vi "Temp Array Gen BAP3B.vi"(8 "error in (no error)":errorcluster, 11 "Temperature Control Parameters":T1={"Start Temp"=0.0, "Temp Step"=5.0, "End Temp"=0.0} {"End Temp" format="%.2f"; "Temp Step" format="%.2f"; "Start Temp" format="%.2f"}) -> (0 "error out":errorcluster, 1 "Temperature Control Parameters Out":T1={"Start Temp"=0.0, "Temp Step"=5.0, "End Temp"=0.0} {"End Temp" format="%.2f"; "Temp Step" format="%.2f"; "Start Temp" format="%.2f"}, 2 "N Temps":i32=6, 3 "Temp Array":dbl[](array[numeric]), 4 "Warning":bool=TRUE)   [LabVIEW 2014]
doc: "Temp Array Gen\n\nCreates an array of temperature given the starting, step, end temperature. This should return an array and the number of temperatures. Takes in consideration inverted limits and steps of zero.\n\nBeverly Abadines\nPHY 350 \nBAP3B"
uses:
  typedefs/temp control params.ctl
panel:
  # "Temp Array Gen"
  # "Beverly Abadines\nPhys 350\nBAP3B"
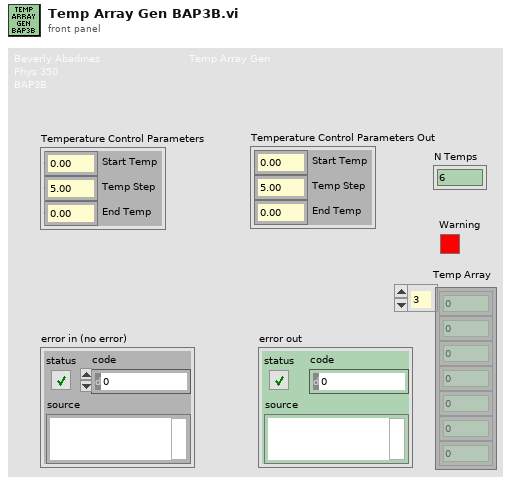
[diagram p1: front panel]
types:
  T1 = typedef "temp control params.ctl" = cluster{"Start Temp":dbl, "Temp Step":dbl, "End Temp":dbl}
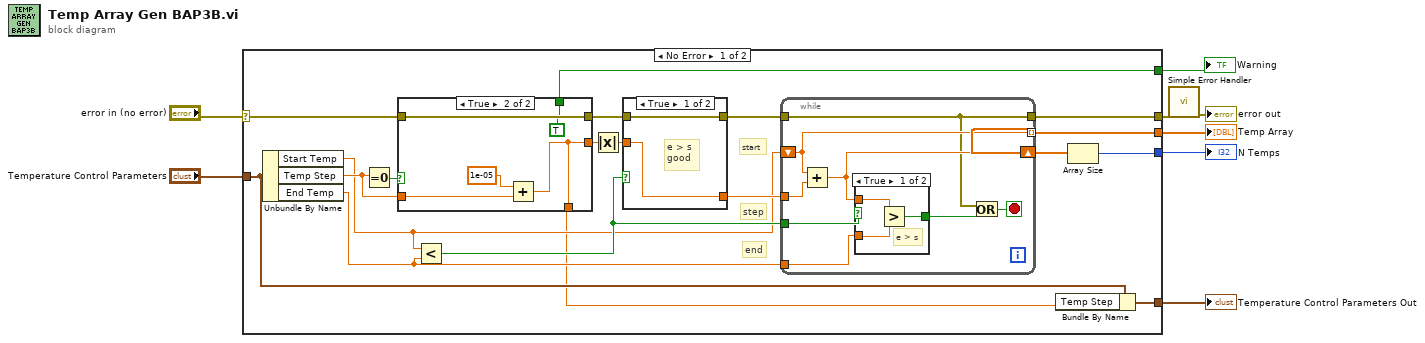
[diagram p0: block diagram]
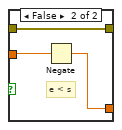
[diagram p2: hidden frame]
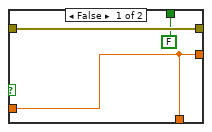
[diagram p3: hidden frame]
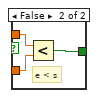
[diagram p4: hidden frame]
diagram:
  n1 = case shown="No Error" "error in (no error)" {
    selector: "error in (no error)" -> [w19 w54]
    tunnel: [w16 w54] -> w5
    tunnel: "Temperature Control Parameters" -> [w11 _]
    tunnel: [w18 _] -> w7
    tunnel: [w17 _] -> w6
    tunnel: [w12 _] -> w2
    tunnel: [w9 _] -> w1
    frame No Error {
      # "end"
      # "step"
      # "start"
      n2 = Unbundle By Name(w11) -> ("Start Temp"=w13:dbl, "Temp Step"=w21:dbl, "End Temp"=w14:dbl)
      n3 = Equal To 0?(x=w21) -> (x = 0?=w20:bool)
      n4 = case shown="True" w20 {
        tunnel: w21 -> [w33 w39]
        tunnel: [w33 w36] -> w22
        tunnel: w19 -> [w34 w37]
        tunnel: [w34 w37] -> w25
        tunnel: [w33 w36] -> w10
        tunnel: [FALSE TRUE] -> w9
        frame False {
        }
        frame True {
          n5 = Add(x=1e-05, y=w39) -> (x+y=w36:dbl)
        }
      }
      n6 = Less?(x=w13, y=w14) -> (x < y?=w24:bool)
      n7 = Absolute Value(x=w22) -> (abs(x)=w23:dbl)
      n8 = case shown="True" w24 {
        tunnel: w23 -> [w28 w31]
        tunnel: [w28 w30] -> w15
        tunnel: w25 -> [w27 w29]
        tunnel: [w27 w29] -> w26
        frame True {
          # "e > s \ngood"
        }
        frame False {
          # "e < s"
          n9 = Negate(x=w31) -> (-x=w30:dbl)
        }
      }
      n10 = while {
        shift-right: [w45] -> _
        shift-left: w13 -> [w47]
        tunnel: [w47] -> w18 mode=indexing
        tunnel: w14 -> [w44]
        tunnel: w15 -> [w46]
        tunnel: w24 -> [w43]
        tunnel: w26 -> [w41]
        tunnel: [w41] -> w16
        stop <- w40 stop-if-true
        n11 = Add(x=w47, y=w46) -> (x+y=w45:dbl)
        n12 = case shown="True" w43 {
          tunnel: w45 -> [w50 w53]
          tunnel: w44 -> [w49 w52]
          tunnel: [w48 w51] -> w42
          frame True {
            # "e > s"
            n13 = Greater?(x=w50, y=w49) -> (0:w48:bool)
          }
          frame False {
            # "e < s"
            n14 = Less?(x=w53, y=w52) -> (x < y?=w51:bool)
          }
        }
        n15 = Or(x=w41, y=w42) -> (x .or. y?=w40:bool)
      }
      n16 = Bundle By Name(cluster=w11, "Temp Step"=w10) -> (w12:T1)
      n17 = Array Size(array=w18) -> (size(s)=w17:i32)
    }
    frame Error {
    }
  }
  "N Temps" <- w6
  "Temp Array" <- w7
  "Temperature Control Parameters Out" <- w2
  "Warning" <- w1
  n18 = call <vilib>:"Simple Error Handler.vi"("error in (no error)"=w5) -> ("error out"=→"error out":errorcluster)  [unwired: 4 in, 4 out]
